vi "Traditional Use of Events for Check Uncheck.vi"() -> ()   [LabVIEW 2017]
panel:
  in  "Listbox 2":i32(listbox)
  in  "stop":bool
  in  "Listbox":i32(listbox)
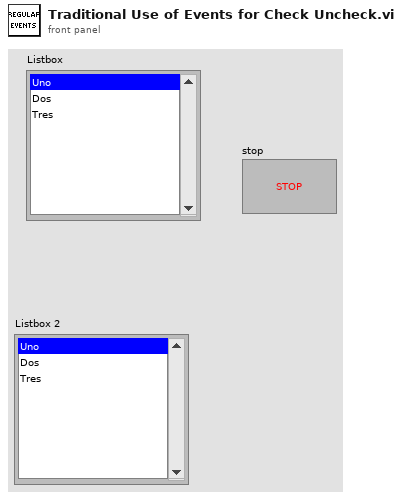
[diagram p1: front panel]
types:
  T1 = typedef "LVPoint32TypeDef.ctl" = cluster{"Horizontal":i32, "Vertical":i32}
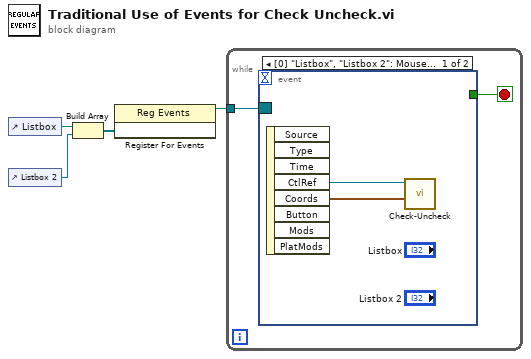
[diagram p0: block diagram]
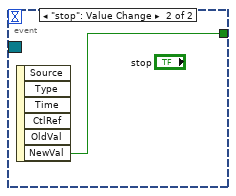
[diagram p2: hidden frame]
diagram:
  n1 = control-ref of="Listbox"() -> (w3:refnum<vi>)
  n2 = control-ref of="Listbox 2"() -> (w2:refnum<vi>)
  n3 = Build Array(w3, w2) -> (w1:refnum<vi>[])
  n4 = register-events(w1) -> (reference out=w4:refnum<event-registration>)  [unwired: 2 in, 1 out]
  n5 = while {
    tunnel: w4 -> [w5]
    stop <- w6 stop-if-true
    n6 = event shown="[0] \"Listbox\", \"Listbox 2\": Mouse Down" {
      selector: w5 -> [_ _]
      dyn-events: _ -> [_ _]
      timeout: _ -> [_ _]
      tunnel: [_ w9] -> w6
      event "Listbox", "Listbox 2": Mouse Down {
        n7 = event-data() -> ("CtlRef"=w8:refnum<vi>, "Coords"=w7:T1)  [unwired: 1 in, 6 out]
        n8 = call "Check-Uncheck.vi"("Coords"=w7, "Listbox Ref"=w8) -> ()  [unwired: 9 in, 1 out]
      }
      event "stop": Value Change {
        n9 = event-data() -> ("NewVal"=w9:bool)  [unwired: 1 in, 5 out]
      }
    }
  }
